vi "Add.vi"() -> ()   [LabVIEW 2024, in "RotateCircularBuffer.Tests.Units.lvlib"]
uses:
  RotateCircularBuffer.Tests.Units.lvlib
  <vilib>/addons/_JKI Toolkits/Caraya/classes/Assert/Assert.lvclass
  <vilib>/addons/_JKI Toolkits/Caraya/classes/Test/Test.lvclass
  RotateCircularBuffer.lvclass
  <vilib>/addons/_JKI Toolkits/Caraya/classes/Assert/Assert True.vi
  TypedCircularBuffer/Type.ctl
  TypedCircularBuffer/TypedCircularBuffer.lvclass
panel:
  in  "expected":i32[](array[numeric])=[1, 2, 3, 4, 5, 6, 7, 8, 9, 10]
  out "Flushed Buffer":T1[](array[typedef])
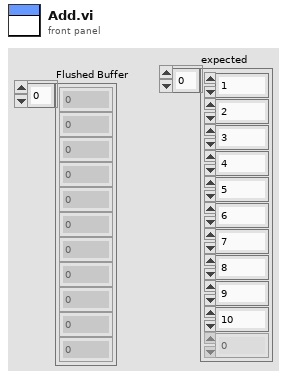
[diagram p1: front panel]
types:
  T1 = typedef "TypedCircularBuffer.lvclass/Type.ctl" = i32
  T2 = typedef "RotateCircularBuffer.lvclass/Type.ctl" = u8
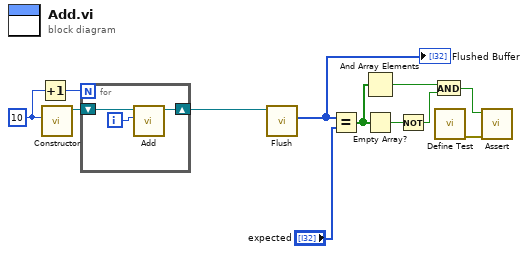
[diagram p0: block diagram]
diagram:
  w4 = u32 10 ("Capacity")
  n1 = Increment(x=w4) -> (x+1=w12:u32)
  n2 = call "Constructor.vi"("Capacity"=w4) -> ("TypedCircularBuffer out"=w3:refnum<class "RotateCircularBuffer.lvclass">)  [unwired: 10 in]
  n3 = for {
    N: w12 -> [_]
    shift-right: [w14] -> w2
    shift-left: w3 -> [w15]
    i -> [w13]
    n4 = call "Add.vi"("Element"=w13, "TypedCircularBuffer in"=w15) -> ("TypedCircularBuffer out"=w14:refnum<class "RotateCircularBuffer.lvclass">)  [unwired: 9 in]
  }
  n5 = call "Flush.vi"("TypedCircularBuffer in"=w2) -> ("Array"=w1:T2[])  [unwired: 9 in, 1 out]
  "Flushed Buffer" <- w1
  n6 = Equal?(x=w1, y="expected") -> (x = y?=w8:bool[])
  n7 = And Array Elements(Boolean array=w8) -> (logical AND=w11:bool)
  n8 = Empty Array?(array=w8) -> (empty?=w10:bool)
  n9 = Not(x=w10) -> (.not. x?=w9:bool)
  n10 = And(x=w11, y=w9) -> (x .and. y?=w7:bool)
  n11 = call <vilib>:"Define Test.vi"() -> ("error out"=w6:errorcluster)  [unwired: 10 in, 1 out]
  n12 = call-poly <vilib>:"Assert.vi"("error in (no error)"=w6, "True?"=w7) -> ()  [unwired: 8 in, 2 out]
